vi "Close.vi"(8 "error in (no error)":errorcluster, 11 "heater_parent in":refnum<class "heater_parent.lvclass">) -> (0 "error out":errorcluster, 3 "heater_parent out":refnum<class "heater_parent.lvclass">)   [LabVIEW 2020, in "polar_bear_plus_drivers.lvlib" / "heater_parent.lvclass"]
doc: "Closes the VISA connection with the instrument."
uses:
  <instrlib>/RxnRover/Driver Polar Bear Plus/heater_parent/heater_parent.lvclass
  <instrlib>/Eurotherm nanodac/Eurotherm nanodac.lvlib
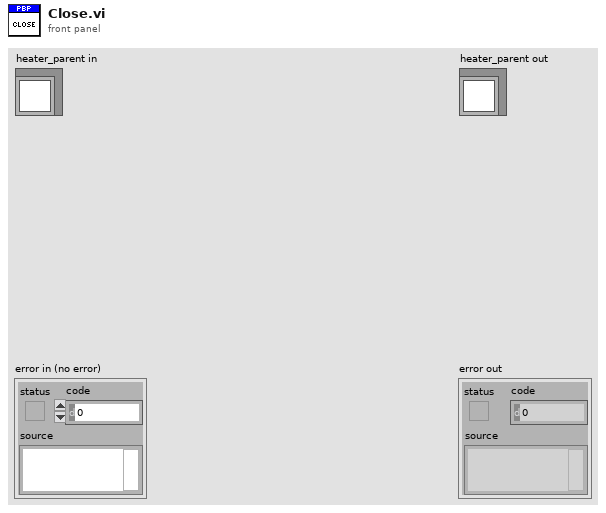
[diagram p1: front panel]
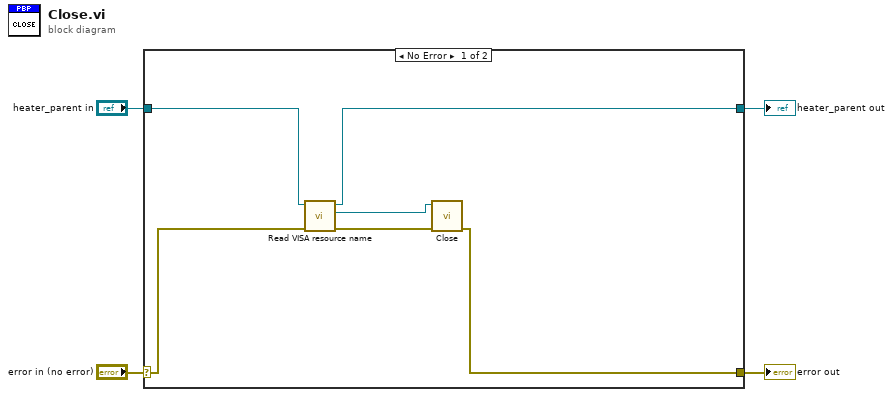
[diagram p0: block diagram]
diagram:
  n1 = case shown="No Error" "error in (no error)" {
    selector: "error in (no error)" -> [w10 w12]
    tunnel: [w5 w12] -> w3
    tunnel: [w8 w11] -> w1
    tunnel: "heater_parent in" -> [w9 w11]
    frame No Error {
      n2 = call-dynamic "Read VISA resource name.vi"("error in (no error)"=w10, "vici_flow_actuator_parent in"=w9) -> ("error out"=w7:errorcluster, "VISA resource name"=w6:refnum<visa-resource-name>, "vici_flow_actuator_parent out"=w8:refnum<class "heater_parent.lvclass">)  [unwired: 7 in]
      n3 = call <instrlib>:"Close.vi"("error in (no error)"=w7, "VISA resource name"=w6) -> ("error out"=w5:errorcluster)  [unwired: 9 in]
    }
    frame Error {
    }
  }
  "error out" <- w3
  "heater_parent out" <- w1
